vi "Check Name.vi"(9 "Name":string, 10 "Msg Attributes in":refnum<data-value>) -> (0 "Error out":errorcluster, 1 "Match":bool, 2 "Msg Attributes out":refnum<data-value>)   [LabVIEW 2020, in "jettl.lvlib"]
uses:
  jettl.lvlib
  Msg/Msg.lvclass
  Msg Input/Msg Input.lvclass
  Msg Output/Msg Output.lvclass
  Relation.ctl
  Teller.ctl
  Msg Attributes.ctl
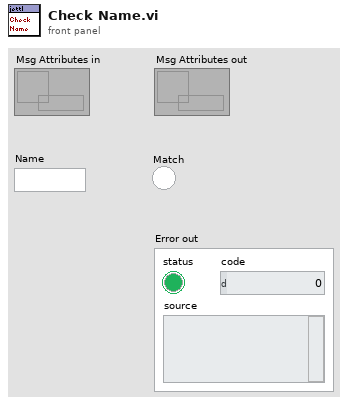
[diagram p1: front panel]
types:
  T1 = typedef "jettl.lvlib/Msg Attributes.ctl" = cluster{"Msg":refnum<class "Msg.lvclass">, "Msg Input":refnum<class "Msg Input.lvclass">, "Msg Output":refnum<class "Msg Output.lvclass">, "Teller":T2}
  T2 = typedef "jettl.lvlib/Teller.ctl" = cluster{"Absolute Time":timestamp, "Relative Time":dbl, "Alias":string, "Relation":T3}
  T3 = typedef "jettl.lvlib/Relation.ctl" = enum16{"Self", "Parent", "Child"}
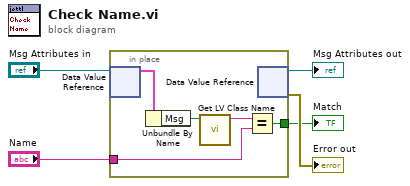
[diagram p0: block diagram]
diagram:
  n1 = in-place {
    in-place-border: [w7] -> w3
    in-place-border: "Name" -> [w6]
    n2 = in-place-dvr #1("Msg Attributes in") -> (w10:T1)  [unwired: 1 out]
    n3 = Unbundle By Name(w10) -> ("Msg"=w9:refnum<class "Msg.lvclass">)
    n4 = call <vilib>:"Get LV Class Name.vi"("object"=w9) -> ("class name"=w8:string)  [unwired: 9 in, 1 out]
    n5 = Equal?(x=w8, y=w6) -> (x = y?=w7:bool)
    n6 = in-place-dvr #1() -> (→"Msg Attributes out":refnum<data-value>, →"Error out":errorcluster)  [unwired: 1 in]
  }
  "Match" <- w3
